vi "Render to String.vi"(7 "Data":cluster{"Key":string, "Value":variant}[](array[cluster]), 8 "Error In":errorcluster, 11 "Render In":refnum<class "Render.lvclass">) -> (0 "Error Out":errorcluster, 2 "Output":string, 3 "Render Out":refnum<class "Render.lvclass">)   [LabVIEW 2018, in "Toolkit.lvlib" / "Render.lvclass"]
uses:
  Render.lvclass
  Writers/String/String.lvclass
  D:/Users/cfield/Code/Field R&D Services/Mustache/trunk/src/Toolkit/Writers/Abstract/Abstract.lvclass
  Writers/String/String.lvclass/String.ctl
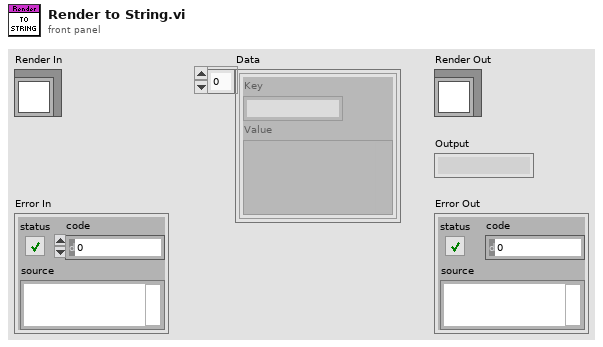
[diagram p1: front panel]
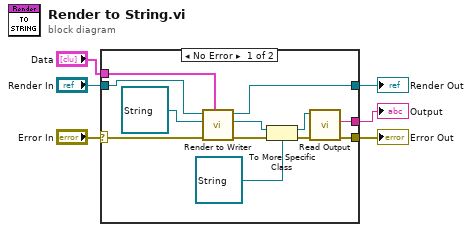
[diagram p0: block diagram]
diagram:
  n1 = case shown="No Error" "Error In" {
    selector: "Error In" -> [w17 w19]
    tunnel: "Render In" -> [w16 w20]
    tunnel: [w15 w20] -> w4
    tunnel: [w14 w19] -> w3
    tunnel: "Data" -> [w12 _]
    tunnel: [w13 _] -> w1
    frame No Error {
      n2 = call "Render to Writer.vi"("Data"=w12, "Error In"=w17, "Writer In"=refnum<class "String.lvclass"> refnum ("Toolkit.lvlib:Writers.lvlib:String.lvclass"), "Render In"=w16) -> ("Error Out"=w18:errorcluster, "Writer Out"=w10:refnum<class "Abstract.lvclass">, "Render Out"=w15:refnum<class "Render.lvclass">)  [unwired: 5 in]
      n3 = To More Specific Class(target class=refnum<class "String.lvclass"> refnum ("Toolkit.lvlib:Writers.lvlib:String.lvclass"), reference=w10, error in=w18) -> (specific class reference=w7:refnum<class "String.lvclass">, error out=w11:errorcluster)
      n4 = call "Read Output.vi"("Error In"=w11, "String In"=w7) -> ("Error Out"=w14:errorcluster, "Output"=w13:string)  [unwired: 7 in, 1 out]
    }
    frame Error {
    }
  }
  "Render Out" <- w4
  "Error Out" <- w3
  "Output" <- w1
